vi "SetTransparancy.vi"(8 "error in (no error)":errorcluster, 10 "Transparency":u8, 11 "WindowFrame in":refnum<class "WindowFrame.lvclass">) -> (0 "error out":errorcluster, 3 "WindowFrame out":refnum<class "WindowFrame.lvclass">)   [LabVIEW 2021, in "WindowFrame.lvlib" / "WindowFrame.lvclass"]
uses:
  WindowFrame.lvclass
  C:/GitHub/ClassUtilities/src/ClassByRef/ClassByRef.lvclass
  ClassUtilities/src/ClassByRef/ClassByRef.lvclass/ClassByRef.ctl
  WindowFrame.lvclass/WindowFrame.ctl
  761eaf14-722b-4189-97e2-c9fceb149270.vi
  ClassUtilities/src/ClassByRef/GetRef.vi
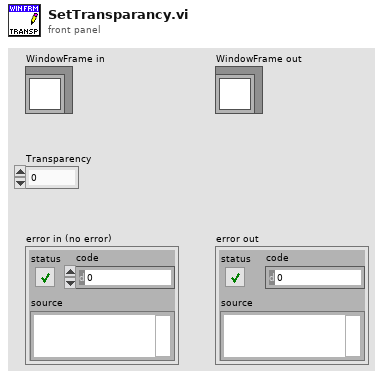
[diagram p1: front panel]
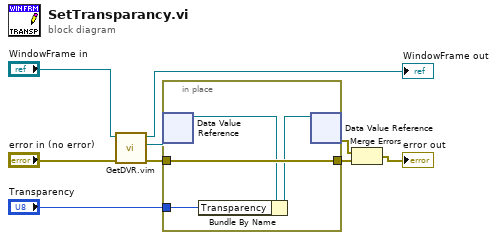
[diagram p0: block diagram]
diagram:
  n1 = call "GetDVR.vim"("error in (no error)"="error in (no error)", "ByRefClass in"="WindowFrame in") -> ("error out"=w4:errorcluster, "DVR"=w3:refnum<data-value>, "ByRefClass out"=→"WindowFrame out":refnum<class "WindowFrame.lvclass">)  [unwired: 7 in]
  n2 = in-place {
    in-place-border: w4 -> [w13]
    in-place-border: [w13] -> w2
    in-place-border: "Transparency" -> [w11]
    n3 = in-place-dvr #1(w3) -> (w12:refnum<class "WindowFrame.lvclass">)  [unwired: 1 out]
    n4 = Bundle By Name(cluster=w12, "Transparency"=w11) -> (w10:refnum<class "WindowFrame.lvclass">)
    n5 = in-place-dvr #1(w10) -> (w1:errorcluster)  [unwired: 1 out]
  }
  n6 = Merge Errors(w1, w2) -> (→"error out":errorcluster)
